vi "Report Filtered Error.vi"(6 "Repeat Time (60s)":dbl=60.0, 8 "error in (no error)":errorcluster, 9 "Message":string, 10 "Context":string, 11 "VolatusAPI in":refnum<class "VolatusAPI.lvclass">) -> (0 "error out":errorcluster, 3 "VolatusAPI out":refnum<class "VolatusAPI.lvclass">)   [LabVIEW 2020, in "Volatus.lvlib" / "VolatusAPI.lvclass"]
uses:
  VolatusAPI.lvclass
  VolatusAPI.lvclass/VolatusAPI.ctl
  Event Level.ctl
  Volatus.lvlib
  Event.ctl
  MessageQ/MessageQ.lvclass
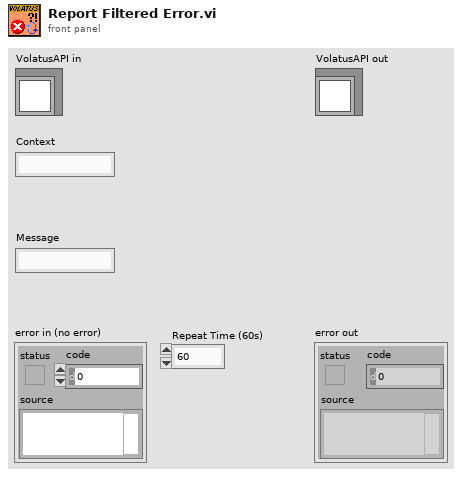
[diagram p1: front panel]
types:
  T1 = typedef "Volatus.lvlib/Event Level.ctl" = enum16{"Debug", "Info", "Warning", "Error"}
  T2 = typedef "Volatus.lvlib/Event.ctl" = cluster{"Time Stamp":timestamp, "Event Level":T1, "Context":string, "Message":string, "Error":errorcluster}
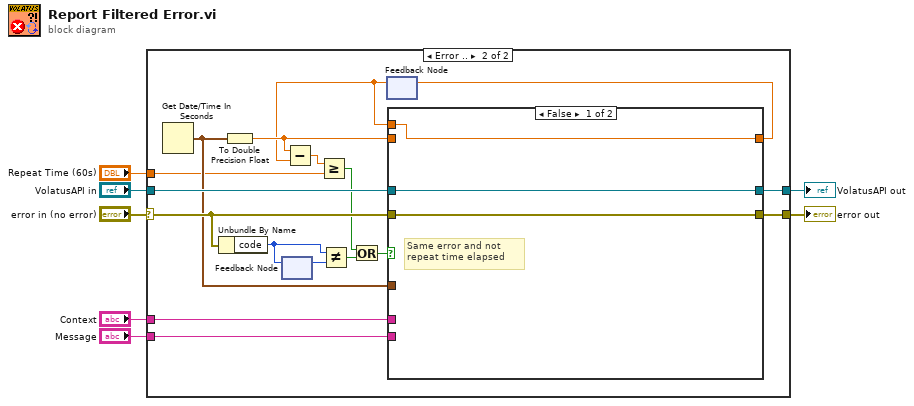
[diagram p0: block diagram]
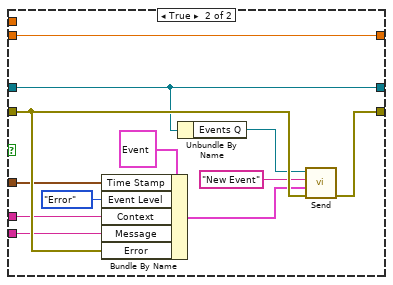
[diagram p3: hidden frame]
diagram:
  n1 = case shown="Error .." "error in (no error)" {
    selector: "error in (no error)" -> [w8 w26]
    tunnel: "VolatusAPI in" -> [w9 w23]
    tunnel: [w9 w19] -> w6
    tunnel: [w8 w22] -> w5
    tunnel: "Context" -> [_ w25]
    tunnel: "Message" -> [_ w24]
    tunnel: "Repeat Time (60s)" -> [_ w14]
    frame No Error {
    }
    frame Error {
      n2 = Get Date/Time In Seconds() -> (seconds since 1Jan1904=w17:timestamp)
      n3 = Unbundle By Name(w26) -> ("code"=w20:i32)
      n4 = To Double Precision Float(number=w17) -> (double precision float=w18:dbl)
      n5 = feedback #1() -> (w21:i32)  [unwired: 1 in]
      n6 = feedback-in #1(w20) -> ()
      n7 = Not Equal?(x=w20, y=w21) -> (x != y?=w13:bool)
      n8 = feedback #2() -> (w10:dbl)  [unwired: 1 in]
      n9 = Subtract(x=w18, y=w10) -> (x-y=w15:dbl)
      n10 = Greater Or Equal?(x=w15, y=w14) -> (x >= y?=w12:bool)
      n11 = Or(x=w12, y=w13) -> (x .or. y?=w11:bool)
      n12 = case shown="False" w11 {
        tunnel: w26 -> [w27 w41]
        tunnel: w25 -> [_ w38]
        tunnel: w24 -> [_ w37]
        tunnel: w23 -> [w29 w32]
        tunnel: [w27 w33] -> w22
        tunnel: [w29 w32] -> w19
        tunnel: w18 -> [_ w30]
        tunnel: w17 -> [_ w31]
        tunnel: [w28 w30] -> w16
        tunnel: w10 -> [w28 _]
        frame False {
          # "Same error and not repeat time elapsed"
        }
        frame True {
          n13 = Bundle By Name(cluster=T2 {"Time Stamp"=timestamp(0 s since 1904-01-01), "Event Level"=enum."Info", "Context"="", "Message"="", "Error"={"status"=FALSE, "code"=0, "source"=""}} ("Event"), "Time Stamp"=w31, "Event Level"=Event_Level."Error", "Context"=w38, "Message"=w37, "Error"=w41) -> (w34:T2)
          n14 = Unbundle By Name(w32) -> ("Events Q"=w36:refnum<class "MessageQ.lvclass">)
          n15 = call "Send.vi"("error in (no error)"=w41, "Data"=w34, "ID"="New Event", "MessageQ in"=w36) -> ("error out"=w33:errorcluster)  [unwired: 6 in, 1 out]
        }
      }
      n16 = feedback-in #2(w16) -> ()
    }
  }
  "error out" <- w5
  "VolatusAPI out" <- w6
